vi "DependencyViewer_Configuration.vi"(8 "error in":errorcluster, 11 "ProjectPath":path) -> (0 "error out":errorcluster)   [LabVIEW 2020]
uses:
  <resource>/Framework/Providers/Open_GDS/DependencyViewer/DependencyChecker/FilterOptions.ctl
  <resource>/Framework/Providers/Open_GDS/SubVIs/GOOP_DependencySettings.ctl
  <resource>/Framework/Providers/Open_GDS/DependencyViewer/DependencyChecker/DependencyConfiguration.ctl
  <vilib>/Utility/sysdir.llb/System Directory Type.ctl
  <resource>/Framework/Providers/Open_GDS/DependencyViewer/DependencyChecker/DependencyChecker.lvlib
panel:
  in  "Max reports to save":u8 min=1
  in  "Close":bool
  in  "SaveChanges":bool
  in  "IgnoreLibrariesInCircularDependencies":bool
  in  "OnlyKeepCircularDepedencies":bool
  in  "Filter Options":T1={"Ignore user.lib"=FALSE, "Ignore vi.lib"=FALSE, "Ignore instr.lib"=FALSE, "FolderToIgnore"=[], "Ignore libraries"=FALSE, "Ignore lvcasses"=FALSE, "Ignore xnodes"=TRUE, "Ignore xcontrols"=TRUE, "Ignore Channel Classes"=TRUE}
  in  "RemoveEvenSubLibraries":bool
  in  "RemoveItemsBelongingToLibraries":bool
  in  "OpenFolder":bool
  in  "EmbedChartScript":bool
  in  "Remove Configuration":bool
  in  "Dependency configuration name":string
  in  "Add Configuration":bool
  in  "_ShowContextHelp":bool
  in  "Help":bool
  in  "Revert":bool
  in  "Update":bool
  out "ProductPicture":picture
  in  "Dependency configurations":i32(listbox) caption="Will show up in the right click menu"
  in  "UseProjectFolder":bool
  in  "Folder to save reports to":path
  # "Dependency Viewer Configuration"
  # "Filter option for configuration"
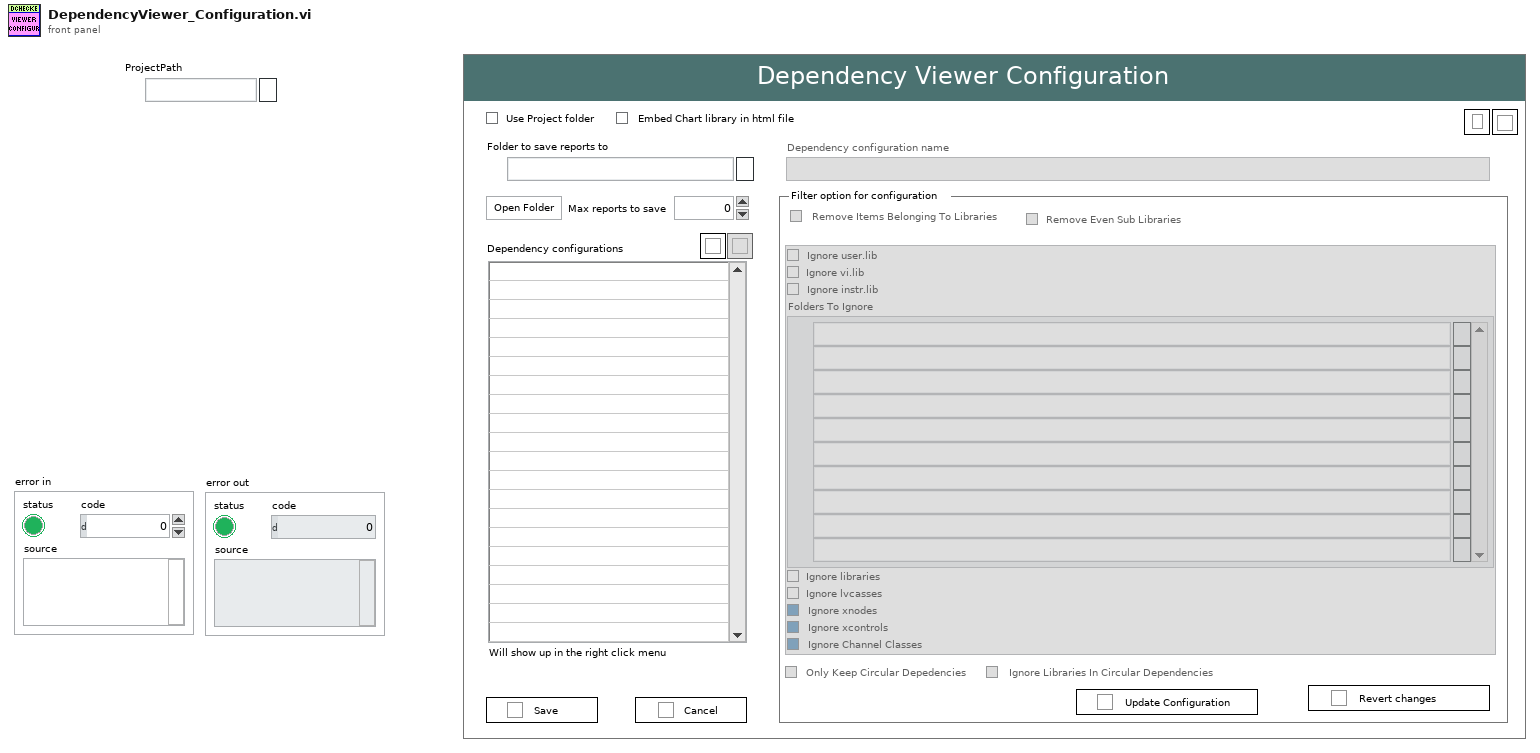
[diagram p1: front panel]
types:
  T1 = typedef "DependencyChecker.lvlib/FilterOptions.ctl" = cluster{"Ignore user.lib":bool, "Ignore vi.lib":bool, "Ignore instr.lib":bool, "FolderToIgnore":path[], "Ignore libraries":bool, "Ignore lvcasses":bool, "Ignore xnodes":bool, "Ignore xcontrols":bool, "Ignore Channel Classes":bool}
  T2 = typedef "System Directory Type.ctl" = i32
  T3 = typedef "GOOP_DependencySettings.ctl" = cluster{"EmbedChartLibraryScript":bool, "Configurations":T4[], "UseProjectFolder":bool, "Folder to save reports to":path, "Max reports to save":u8}
  T4 = typedef "DependencyChecker.lvlib/DependencyConfiguration.ctl" = cluster{"Name":string, "RemoveItemsBelongingToLibraries":bool, "RemoveEvenSubLibraries":bool, "FilterOptions":T1, "OnlyKeepCircularDepedencies":bool, "IgnoreLibrariesInCircularDependencies":bool}
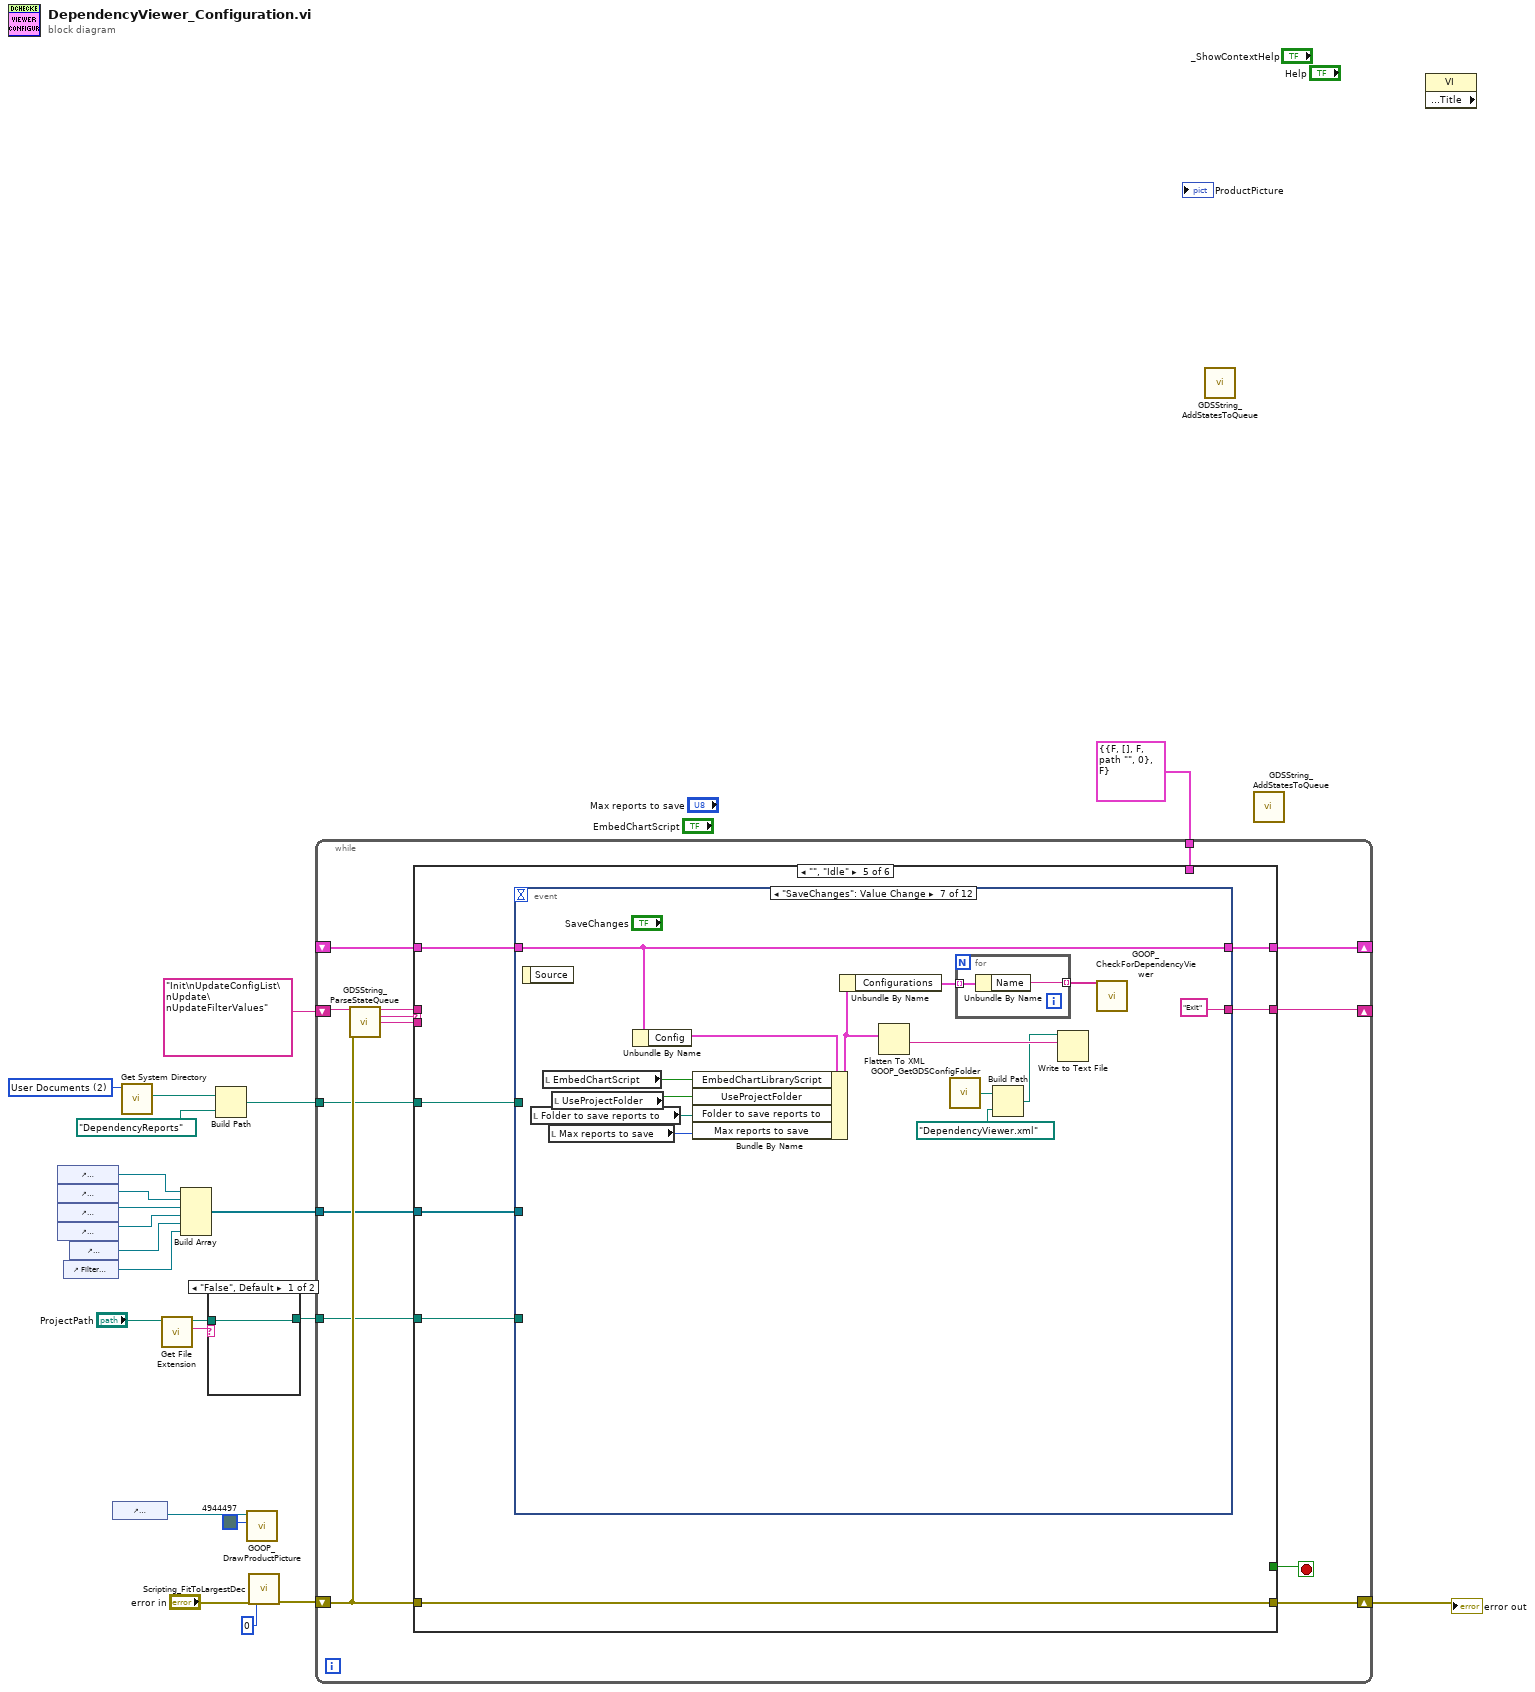
[diagram p0: block diagram]
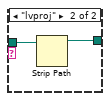
[diagram p2: hidden frame]
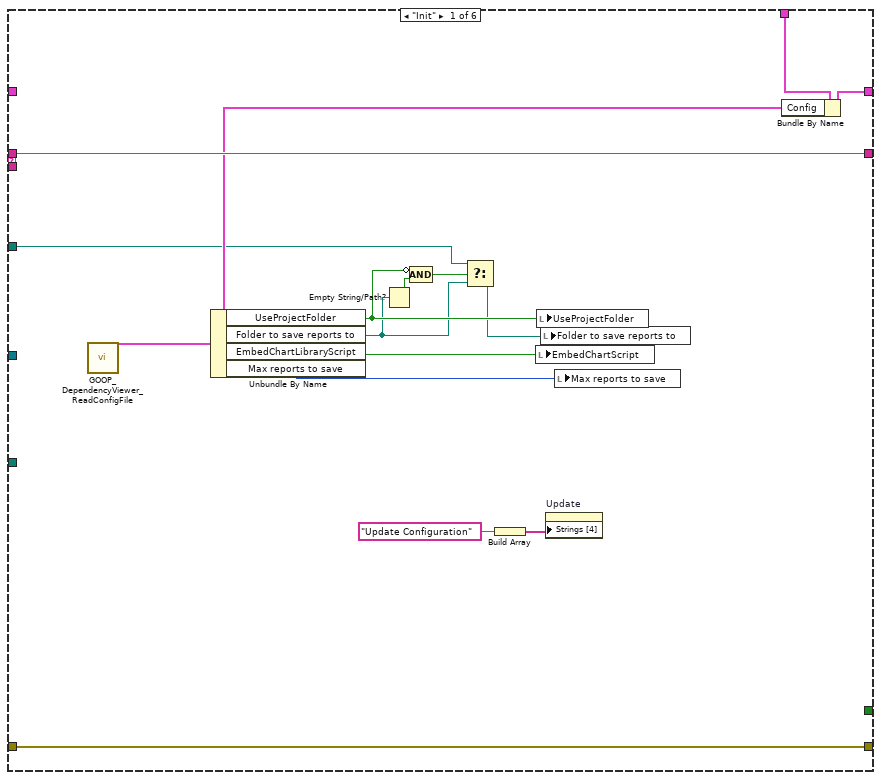
[diagram p3: hidden frame]
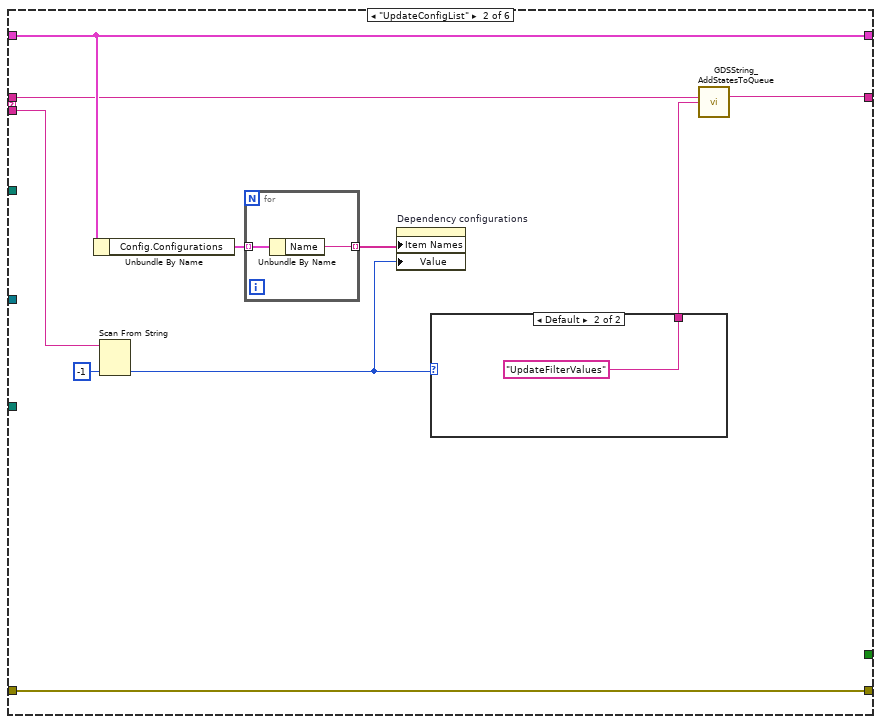
[diagram p4: hidden frame]
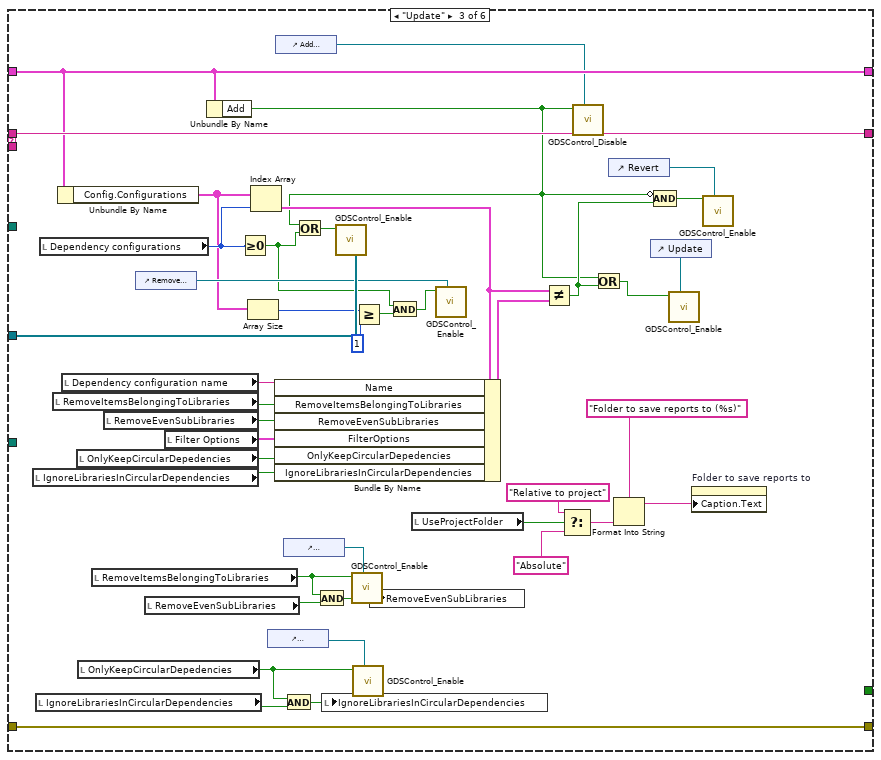
[diagram p6: hidden frame]
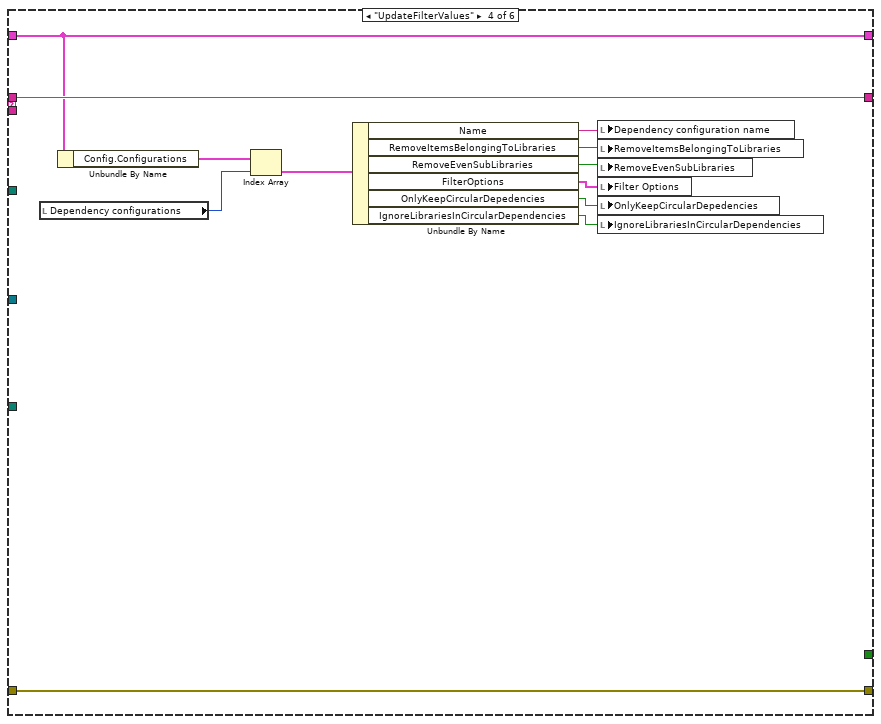
[diagram p7: hidden frame]
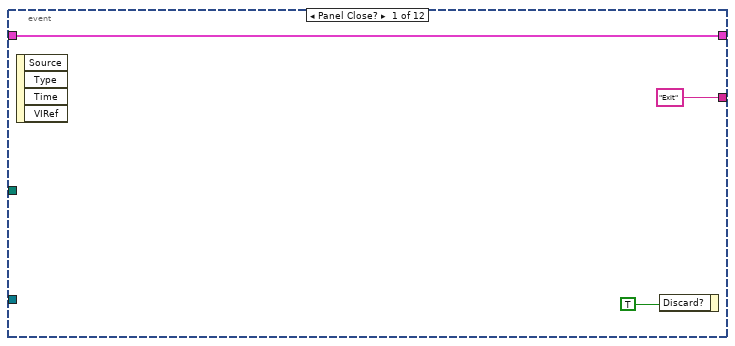
[diagram p8: hidden frame]
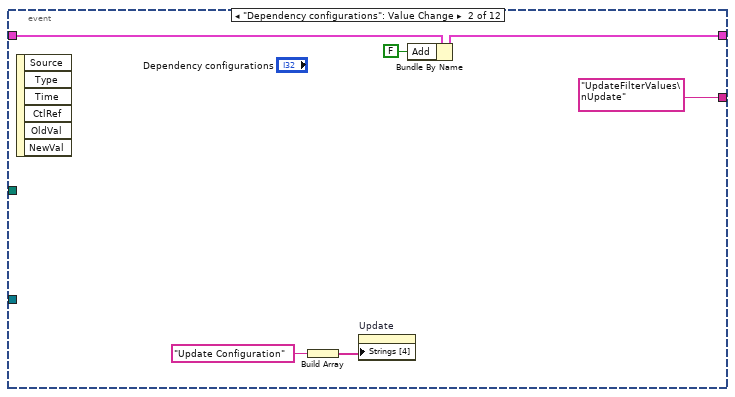
[diagram p9: hidden frame]
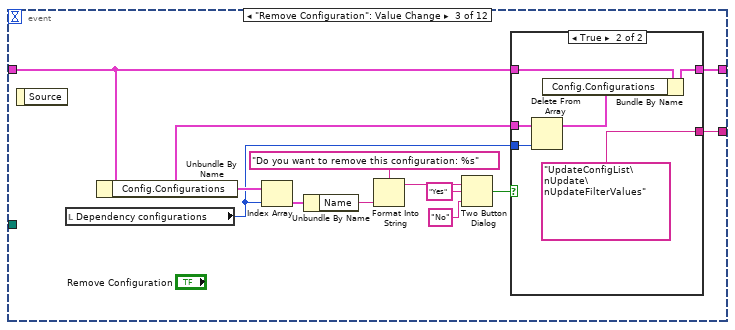
[diagram p10: hidden frame]
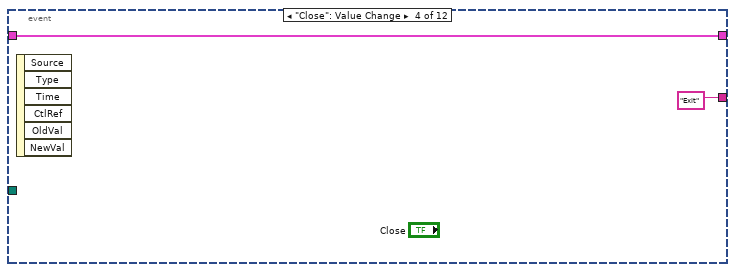
[diagram p12: hidden frame]
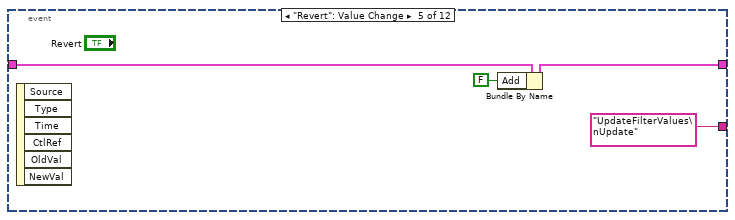
[diagram p13: hidden frame]
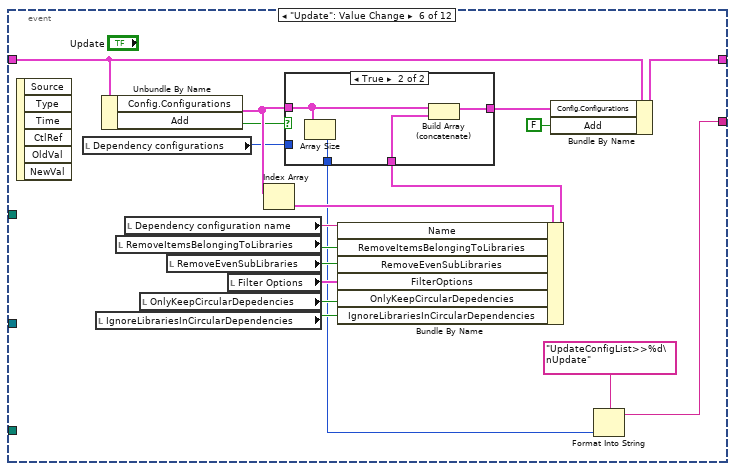
[diagram p14: hidden frame]
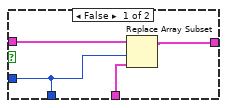
[diagram p15: hidden frame]
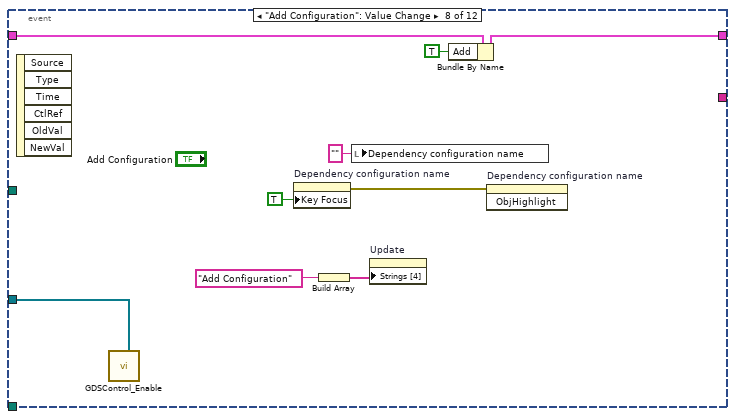
[diagram p16: hidden frame]
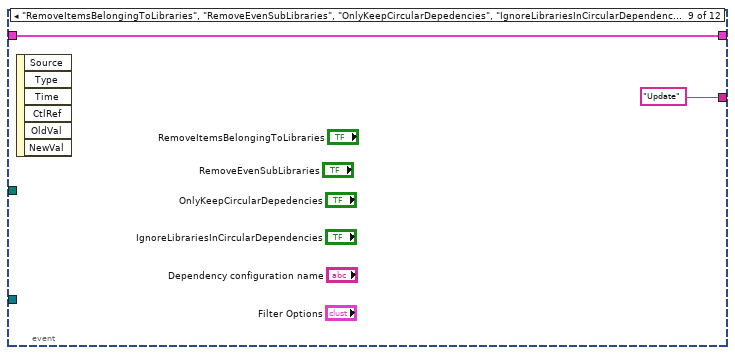
[diagram p17: hidden frame]
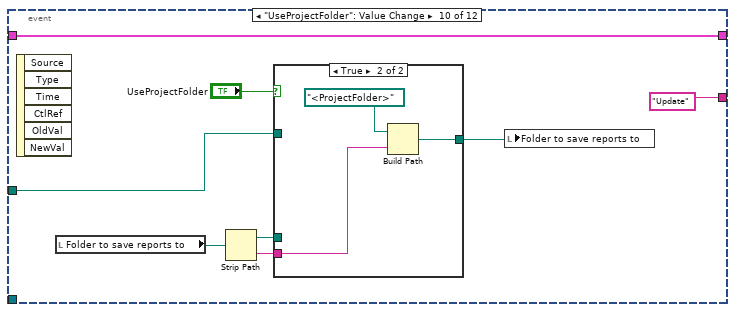
[diagram p18: hidden frame]
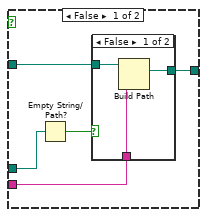
[diagram p19: hidden frame]
diagram:
  w8 = T2 2 items=["User Home"=0, "User Desktop"=1, "User Documents"=2, "User Application Data"=3, "User Preferences"=4, "User Temporary"=5, "Public Documents"=6, "Public Application Data"=7, "Public Preferences"=8, "Public Cache"=13, "System Core Libraries"=9, "System Installed Libraries"=10, "Application Files"=11, "Boot Volume Root"=12] ("system directory type")
  n1 = control-ref of="IgnoreLibrariesInCircularDependencies"() -> (w17:refnum<vi>)
  n2 = control-ref of="OnlyKeepCircularDepedencies"() -> (w16:refnum<vi>)
  n3 = control-ref of="RemoveEvenSubLibraries"() -> (w15:refnum<vi>)
  n4 = control-ref of="RemoveItemsBelongingToLibraries"() -> (w14:refnum<vi>)
  n5 = control-ref of="Filter Options"() -> (w12:refnum<vi>)
  n6 = control-ref of="Dependency configuration name"() -> (w13:refnum<vi>)
  n7 = control-ref of="ProductPicture"() -> (w22:refnum<vi>)
  n8 = call <vilib>:"Get System Directory.vi"("system directory type"=w8) -> ("system directory"=w7:path)  [unwired: 10 in]
  n9 = call <vilib>:"Get File Extension.vi"("file"="ProjectPath") -> ("lowercase file extension"=w3:string, "dup file"=w2:path)  [unwired: 6 in, 3 out]
  n10 = Build Array(w17, w16, w15, w14, w13, w12) -> (w11:refnum<vi>[])
  n11 = case shown="\"False\", Default" w3 {
    tunnel: w2 -> [w24 w26]
    tunnel: [w24 w25] -> w1
    frame "False", Default {
    }
    frame "lvproj" {
      n12 = Strip Path(path=w26) -> (stripped path=w25:path)  [unwired: 1 out]
    }
  }
  n13 = Build Path(base path=w7, name or relative path=path "DependencyReports") -> (appended path=w5:path)
  n14 = call <resource>:"GOOP_DrawProductPicture.vi"("BAckground ColorPane Color"=u32 4944497, "ProductPictureControl"=w22) -> ()  [unwired: 9 in, 1 out]
  n15 = call <resource>:"Scripting_FitToLargestDec.vi"("error in (no error)"="error in", "border spacing (2 px)"=0) -> ("error out"=w18:errorcluster)  [unwired: 4 in, 1 out]
  n16 = while {
    shift-right: [w35] -> _
    shift-left: "Init\nUpdateConfigList\nUpdate\nUpdateFilterValues" -> [w40]
    shift-right: [w37] -> w20
    shift-left: w18 -> [w38]
    tunnel: cluster{"Config":T3, "Add":bool} {"Config"={"EmbedChartLibraryScript"=FALSE, "Configurations"=[], "UseProjectFolder"=FALSE, "Folder to save reports to"=path "", "Max reports to save"=0}, "Add"=FALSE} -> [w33]
    shift-right: [w32] -> _
    shift-left: _ -> [w31]
    tunnel: w11 -> [w29]
    tunnel: w5 -> [w28]
    tunnel: w1 -> [w27]
    stop <- w34 stop-if-true
    n17 = call <resource>:"GDSString_ParseStateQueue.vi"("State Queue"=w40, "Error In (no error)"=w38) -> ("Remaining States"=w36:string, "Current State"=w39:string, "Arguments"=w30:string)  [unwired: 9 in, 2 out]
    n18 = case shown="\"\", \"Idle\"" w39 {
      tunnel: w38 -> [w55 w65 w101 w121 w129 w265]
      tunnel: [w55 w65 w101 w121 w129 w265] -> w37
      tunnel: [w54 w58 w102 w122 w126 w267] -> w35
      tunnel: w36 -> [w54 w59 w102 w122 _ w267]
      tunnel: [_ _ _ _ _ TRUE] -> w34
      tunnel: w33 -> [w53 _ _ _ _ _]
      tunnel: [w52 w63 w83 w120 w127 w264] -> w32
      tunnel: w31 -> [_ w63 w83 w120 w128 w264]
      tunnel: w30 -> [_ w61 _ _ _ _]
      tunnel: w29 -> [_ _ w99 _ w123 _]
      tunnel: w28 -> [w41 _ _ _ w125 _]
      tunnel: w27 -> [_ _ _ _ w124 _]
      frame "Init" {
        n19 = call <resource>:"GOOP_DependencyViewer_ReadConfigFile.vi"() -> ("Config"=w51:T3)  [unwired: 11 in]
        n20 = Unbundle By Name(w51) -> ("UseProjectFolder"=w46:bool, "Folder to save reports to"=w43:path, "EmbedChartLibraryScript"=w50:bool, "Max reports to save"=w47:u8)
        n21 = Empty String/Path?(string/path=w43) -> (empty?=w45:bool)
        n22 = Compound Arithmetic op=AND(invert w46, w45) -> (w44:bool)
        n23 = Select(t=w41, s=w44, f=w43) -> (s? t:f=w42:path)
        n24 = Build Array("Update Configuration") -> (w49:string[])
        n25 = local write "EmbedChartScript"(w50) -> ()
        n26 = local write "UseProjectFolder"(w46) -> ()
        n27 = local write "Folder to save reports to"(w42) -> ()
        n28 = property on="Update" class="Bool"("Strings [4]"=w49) -> ()  [unwired: 2 in, 2 out]
        n29 = local write "Max reports to save"(w47) -> ()
        n30 = Bundle By Name(cluster=w53, "Config"=w51) -> (w52:cluster{"Config":T3, "Add":bool})
      }
      frame "UpdateConfigList" {
        n31 = Unbundle By Name(w63) -> ("Config.Configurations"=w64:T4[])
        n32 = Scan From String(input string=w61, default 1=-1 ("default value 1")) -> (output 1=w57:i32)  [unwired: 3 in, 3 out]
        n33 = for {
          tunnel: w64 -> [w68] mode=indexing
          tunnel: [w67] -> w62 mode=indexing
          n34 = Unbundle By Name(w68) -> ("Name"=w67:string)
        }
        n35 = property on="Dependency configurations" class="LstBox (strict)"("Item Names"=w62, "Value"=w57) -> ()  [unwired: 2 in, 2 out]
        n36 = case shown="Default" w57 {
          tunnel: [_ "UpdateFilterValues"] -> w56
          frame -1 {
          }
          frame Default {
          }
        }
        n37 = call <resource>:"GDSString_AddStatesToQueue.vi"("State(s) in (\"\")"=w59, "State(s) at Back (\"\")"=w56) -> ("States Out"=w58:string)  [unwired: 13 in]
      }
      frame "Update" {
        n38 = local read "IgnoreLibrariesInCircularDependencies"() -> (w92:bool)
        n39 = local read "IgnoreLibrariesInCircularDependencies"() -> (w104:bool)
        n40 = local read "Dependency configurations"() -> (w100:i32)
        n41 = local read "RemoveItemsBelongingToLibraries"() -> (w96:bool)
        n42 = Unbundle By Name(w83) -> ("Config.Configurations"=w89:T4[])
        n43 = local read "Dependency configuration name"() -> (w97:string)
        n44 = local read "OnlyKeepCircularDepedencies"() -> (w93:bool)
        n45 = local read "OnlyKeepCircularDepedencies"() -> (w105:bool)
        n46 = local read "RemoveItemsBelongingToLibraries"() -> (w108:bool)
        n47 = local read "RemoveEvenSubLibraries"() -> (w95:bool)
        n48 = control-ref of="Remove Configuration"() -> (w98:refnum<vi>)
        n49 = local read "RemoveEvenSubLibraries"() -> (w109:bool)
        n50 = local read "Filter Options"() -> (w94:T1)
        n51 = Unbundle By Name(w83) -> ("Add"=w70:bool)
        n52 = Greater Or Equal To 0?(x=w100) -> (x >= 0?=w74:bool)
        n53 = Array Size(array=w89) -> (size(s)=w88:i32)
        n54 = Index Array(array=w89, index=w100) -> (element=w90:T4)
        n55 = control-ref of="IgnoreLibrariesInCircularDependencies"() -> (w106:refnum<vi>)
        n56 = Bundle By Name(cluster=w90, "Name"=w97, "RemoveItemsBelongingToLibraries"=w96, "RemoveEvenSubLibraries"=w95, "FilterOptions"=w94, "OnlyKeepCircularDepedencies"=w93, "IgnoreLibrariesInCircularDependencies"=w92) -> (w91:T4)
        n57 = control-ref of="Add Configuration"() -> (w69:refnum<vi>)
        n58 = control-ref of="RemoveEvenSubLibraries"() -> (w110:refnum<vi>)
        n59 = And(x=w105, y=w104) -> (x .and. y?=w103:bool)
        n60 = Or(x=w70, y=w74) -> (x .or. y?=w73:bool)
        n61 = And(x=w108, y=w109) -> (x .and. y?=w107:bool)
        n62 = local write "IgnoreLibrariesInCircularDependencies"(w103) -> ()
        n63 = call <resource>:"GDSControl_Enable.vi"("ManyControls"=w99, "Enable(True)"=w73) -> ()  [unwired: 9 in, 1 out]
        n64 = call <resource>:"GDSControl_Enable.vi"("ControlRefnum(IgnoreIfNotWired)"=w110, "Enable(True)"=w108) -> ()  [unwired: 9 in, 1 out]
        n65 = call <resource>:"GDSControl_Enable.vi"("ControlRefnum(IgnoreIfNotWired)"=w106, "Enable(True)"=w105) -> ()  [unwired: 9 in, 1 out]
        n66 = Greater Or Equal?(x=w88, y=1) -> (x >= y?=w86:bool)
        n67 = local write "RemoveEvenSubLibraries"(w107) -> ()
        n68 = And(x=w74, y=w86) -> (x .and. y?=w85:bool)
        n69 = local read "UseProjectFolder"() -> (w79:bool)
        n70 = call <resource>:"GDSControl_Enable.vi"("ControlRefnum(IgnoreIfNotWired)"=w98, "Enable(True)"=w85) -> ()  [unwired: 9 in, 1 out]
        n71 = Not Equal?(x=w90, y=w91) -> (x != y?=w72:bool)
        n72 = Select(t="Relative to project", s=w79, f="Absolute") -> (s? t:f=w78:string)
        n73 = call <resource>:"GDSControl_Disable.vi"("ControlRefnum(IgnoreIfNotWired)"=w69, "Disasble(True)"=w70) -> ()  [unwired: 9 in, 1 out]
        n74 = Or(x=w70, y=w72) -> (x .or. y?=w71:bool)
        n75 = control-ref of="Revert"() -> (w81:refnum<vi>)
        n76 = Format Into String(format string="Folder to save reports to (%s)", w78) -> (resulting string=w77:string)  [unwired: 2 in, 1 out]
        n77 = control-ref of="Update"() -> (w84:refnum<vi>)
        n78 = Compound Arithmetic op=AND(invert w70, w72) -> (w82:bool)
        n79 = call <resource>:"GDSControl_Enable.vi"("ControlRefnum(IgnoreIfNotWired)"=w84, "Enable(True)"=w71) -> ()  [unwired: 9 in, 1 out]
        n80 = property on="Folder to save reports to" class="Path"("Caption.Text"=w77) -> ()  [unwired: 2 in, 2 out]
        n81 = call <resource>:"GDSControl_Enable.vi"("ControlRefnum(IgnoreIfNotWired)"=w81, "Enable(True)"=w82) -> ()  [unwired: 9 in, 1 out]
      }
      frame "UpdateFilterValues" {
        n82 = local read "Dependency configurations"() -> (w118:i32)
        n83 = Unbundle By Name(w120) -> ("Config.Configurations"=w119:T4[])
        n84 = Index Array(array=w119, index=w118) -> (element=w117:T4)
        n85 = Unbundle By Name(w117) -> ("Name"=w116:string, "RemoveItemsBelongingToLibraries"=w115:bool, "RemoveEvenSubLibraries"=w114:bool, "FilterOptions"=w113:T1, "OnlyKeepCircularDepedencies"=w112:bool, "IgnoreLibrariesInCircularDependencies"=w111:bool)
        n86 = local write "Dependency configuration name"(w116) -> ()
        n87 = local write "RemoveItemsBelongingToLibraries"(w115) -> ()
        n88 = local write "RemoveEvenSubLibraries"(w114) -> ()
        n89 = local write "Filter Options"(w113) -> ()
        n90 = local write "OnlyKeepCircularDepedencies"(w112) -> ()
        n91 = local write "IgnoreLibrariesInCircularDependencies"(w111) -> ()
      }
      frame "", "Idle" {
        n92 = event shown="[6] \"SaveChanges\": Value Change" {
          selector: _ -> [_ _ _ _ _ _ _ _ _ _ _ _]
          dyn-events: _ -> [_ _ _ _ _ _ _ _ _ _ _ _]
          timeout: _ -> [_ _ _ _ _ _ _ _ _ _ _ _]
          tunnel: w128 -> [w132 w137 w141 w159 w163 w175 w202 w214 w216 w224 w244 w260]
          tunnel: [w132 w134 w143 w159 w161 w174 w202 w210 w216 w224 w244 w260] -> w127
          tunnel: ["Exit" "UpdateFilterValues\nUpdate" w139 "Exit" "UpdateFilterValues\nUpdate" w165 "Exit" _ "Update" "Update" _ _] -> w126
          tunnel: w125 -> [_ _ _ _ _ _ _ _ _ w218 _ _]
          tunnel: w124 -> [_ _ _ _ _ _ _ _ _ _ w239 _]
          tunnel: w123 -> [_ _ _ _ _ _ _ w211 _ _ _ _]
          event Panel Close? {
            n93 = event-data() -> ()  [unwired: 1 in, 4 out]
            n94 = event-data("Discard?"=TRUE) -> ()  [unwired: 1 in, 1 out]
          }
          event "Dependency configurations": Value Change {
            n95 = event-data() -> ()  [unwired: 1 in, 6 out]
            n96 = Build Array("Update Configuration") -> (w136:string[])
            n97 = property on="Update" class="Bool"("Strings [4]"=w136) -> ()  [unwired: 2 in, 2 out]
            n98 = Bundle By Name(cluster=w137, "Add"=FALSE) -> (w134:cluster{"Config":T3, "Add":bool})
          }
          event "Remove Configuration": Value Change {
            n99 = event-data() -> ()  [unwired: 1 in, 1 out]
            n100 = local read "Dependency configurations"() -> (w140:i32)
            n101 = Unbundle By Name(w141) -> ("Config.Configurations"=w142:T4[])
            n102 = Index Array(array=w142, index=w140) -> (element=w150:T4)
            n103 = Unbundle By Name(w150) -> ("Name"=w148:string)
            n104 = Format Into String(format string="Do you want to remove this configuration: %s", w148) -> (resulting string=w147:string)  [unwired: 2 in, 1 out]
            n105 = Two Button Dialog(message=w147, 1:"No" ("T button name (\"OK\")"), 2:"Yes" ("T button name (\"OK\")")) -> (T button?=w144:bool)
            n106 = case shown="True" w144 {
              tunnel: [w151 w154] -> w143
              tunnel: w142 -> [_ w157]
              tunnel: w141 -> [w151 w156]
              tunnel: w140 -> [_ w153]
              tunnel: [_ "UpdateConfigList\nUpdate\nUpdateFilterValues"] -> w139
              frame False {
              }
              frame True {
                n107 = Delete From Array(array=w157, index=w153) -> (array with subset deleted=w155:T4[])  [unwired: 1 in, 1 out]
                n108 = Bundle By Name(cluster=w156, "Config.Configurations"=w155) -> (w154:cluster{"Config":T3, "Add":bool})
              }
            }
          }
          event "Close": Value Change {
            n109 = event-data() -> ()  [unwired: 1 in, 6 out]
          }
          event "Revert": Value Change {
            n110 = event-data() -> ()  [unwired: 1 in, 6 out]
            n111 = Bundle By Name(cluster=w163, "Add"=FALSE) -> (w161:cluster{"Config":T3, "Add":bool})
          }
          event "Update": Value Change {
            n112 = event-data() -> ()  [unwired: 1 in, 6 out]
            n113 = local read "Dependency configurations"() -> (w168:i32)
            n114 = local read "IgnoreLibrariesInCircularDependencies"() -> (w176:bool)
            n115 = Unbundle By Name(w175) -> ("Config.Configurations"=w171:T4[], "Add"=w169:bool)
            n116 = local read "RemoveItemsBelongingToLibraries"() -> (w180:bool)
            n117 = local read "Dependency configuration name"() -> (w181:string)
            n118 = local read "OnlyKeepCircularDepedencies"() -> (w177:bool)
            n119 = local read "RemoveEvenSubLibraries"() -> (w179:bool)
            n120 = local read "Filter Options"() -> (w178:T1)
            n121 = Index Array(array=w171) -> (element=w170:T4)  [unwired: 1 in]
            n122 = Bundle By Name(cluster=w170, "Name"=w181, "RemoveItemsBelongingToLibraries"=w180, "RemoveEvenSubLibraries"=w179, "FilterOptions"=w178, "OnlyKeepCircularDepedencies"=w177, "IgnoreLibrariesInCircularDependencies"=w176) -> (w173:T4)
            n123 = case shown="True" w169 {
              tunnel: w173 -> [w183 w189]
              tunnel: [w184 w188] -> w172
              tunnel: w171 -> [w185 w187]
              tunnel: w168 -> [w182 _]
              tunnel: [w182 w186] -> w164
              frame False {
                n124 = Replace Array Subset(array=w185, new element=w183, index=w182) -> (w184:T4[])
              }
              frame True {
                n125 = Array Size(array=w187) -> (size(s)=w186:i32)
                n126 = Build Array (concatenate)(w187, w189) -> (w188:T4[])
              }
            }
            n127 = Bundle By Name(cluster=w175, "Config.Configurations"=w172, "Add"=FALSE) -> (w174:cluster{"Config":T3, "Add":bool})
            n128 = Format Into String(format string="UpdateConfigList>>%d\nUpdate", w164) -> (resulting string=w165:string)  [unwired: 2 in, 1 out]
          }
          event "SaveChanges": Value Change {
            n129 = event-data() -> ()  [unwired: 1 in, 1 out]
            n130 = local read "Folder to save reports to"() -> (w191:path)
            n131 = local read "EmbedChartScript"() -> (w193:bool)
            n132 = local read "Max reports to save"() -> (w190:u8)
            n133 = local read "UseProjectFolder"() -> (w192:bool)
            n134 = Unbundle By Name(w202) -> ("Config"=w197:T3)
            n135 = Bundle By Name(cluster=w197, "EmbedChartLibraryScript"=w193, "UseProjectFolder"=w192, "Folder to save reports to"=w191, "Max reports to save"=w190) -> (w196:T3)
            n136 = Unbundle By Name(w196) -> ("Configurations"=w195:T4[])
            n137 = Flatten To XML(6:w196) -> (2:w199:string)
            n138 = call <resource>:"GOOP_GetGDSConfigFolder.vi"() -> ("GDSFolderPath"=w201:path)
            n139 = for {
              tunnel: [w205] -> w194 mode=indexing
              tunnel: w195 -> [w204] mode=indexing
              n140 = Unbundle By Name(w204) -> ("Name"=w205:string)
            }
            n141 = Build Path(base path=w201, name or relative path=path "DependencyViewer.xml") -> (appended path=w198:path)
            n142 = Write to Text File(file (use dialog)=w198, text=w199) -> ()  [unwired: 2 in, 3 out]
            n143 = call <resource>:"GOOP_CheckForDependencyViewer.vi"("Configurations"=w194) -> ()  [unwired: 8 in, 3 out]
          }
          event "Add Configuration": Value Change {
            n144 = event-data() -> ()  [unwired: 1 in, 6 out]
            n145 = call <resource>:"GDSControl_Enable.vi"("ManyControls"=w211) -> ()  [unwired: 10 in, 1 out]
            n146 = property on="Dependency configuration name" class="Str"("Key Focus"=TRUE ("Add")) -> (error out=w206:errorcluster)  [unwired: 2 in, 1 out]
            n147 = Build Array("Add Configuration") -> (w213:string[])
            n148 = local write "Dependency configuration name"("" ("Dependency configuration name")) -> ()
            n149 = property on="Update" class="Bool"("Strings [4]"=w213) -> ()  [unwired: 2 in, 2 out]
            n150 = Bundle By Name(cluster=w214, "Add"=TRUE) -> (w210:cluster{"Config":T3, "Add":bool})
            n151 = invoke on="Dependency configuration name" class="Str" method="ObjHighlight"(error in=w206) -> ()  [unwired: 2 in, 3 out]
          }
          event "RemoveItemsBelongingToLibraries", "RemoveEvenSubLibraries", "OnlyKeepCircularDepedencies", "IgnoreLibrariesInCircularDependencies", "Dependency configuration name": Value Change {
            n152 = event-data() -> ()  [unwired: 1 in, 6 out]
          }
          event "UseProjectFolder": Value Change {
            n153 = event-data() -> ()  [unwired: 1 in, 6 out]
            n154 = local read "Folder to save reports to"() -> (w221:path)
            n155 = Strip Path(path=w221) -> (stripped path=w217:path, name=w220:string)
            n156 = case shown="True" "UseProjectFolder" {
              tunnel: w220 -> [w225 w235]
              tunnel: [w226 w234] -> w219
              tunnel: w218 -> [w229 _]
              tunnel: w217 -> [w228 _]
              frame False {
                n157 = Empty String/Path?(string/path=w228) -> (empty?=w227:bool)
                n158 = case shown="False" w227 {
                  tunnel: w229 -> [w232 w233]
                  tunnel: [w230 w233] -> w226
                  tunnel: w225 -> [w231 _]
                  frame False {
                    n159 = Build Path(base path=w232, name or relative path=w231) -> (appended path=w230:path)
                  }
                  frame True {
                  }
                }
              }
              frame True {
                n160 = Build Path(base path=path "<ProjectFolder>", name or relative path=w235) -> (appended path=w234:path)
              }
            }
            n161 = local write "Folder to save reports to"(w219) -> ()
          }
          event "OpenFolder": Value Change {
            n162 = event-data() -> ()  [unwired: 1 in, 6 out]
            n163 = local read "Folder to save reports to"() -> (w241:path)
            n164 = local read "UseProjectFolder"() -> (w242:bool)
            n165 = case shown="True" w242 {
              tunnel: w241 -> [w245 w249]
              tunnel: [w245 w246] -> w238
              tunnel: w239 -> [_ w248]
              frame False {
              }
              frame True {
                n166 = Strip Path(path=w249) -> (name=w247:string)  [unwired: 1 out]
                n167 = Build Path(base path=w248, name or relative path=w247) -> (appended path=w246:path)
              }
            }
            n168 = call <vilib>:"Create Directory Recursive.vi"("directory"=w238) -> ("directory copy"=w237:path)  [unwired: 4 in, 2 out]
            n169 = Format Into String(format string="explorer \"%s\"", w237) -> (resulting string=w240:string)  [unwired: 2 in, 1 out]
            n170 = call <vilib>:"System Exec.vi"("command line"=w240) -> ()  [unwired: 7 in, 4 out]
          }
          event "Folder to save reports to": Value Change {
            n171 = event-data() -> ()  [unwired: 1 in, 6 out]
            n172 = Path Type(1:"Folder to save reports to") -> (0:w257:i16)
            n173 = Strip Path(path="Folder to save reports to") -> (name=w259:string)  [unwired: 1 out]
            n174 = Equal?(x=w257, y=i16 1) -> (x = y?=w253:bool)
            n175 = Match Pattern(string=w259, regular expression="<") -> (offset past match=w255:i32)  [unwired: 1 in, 3 out]
            n176 = Greater Or Equal To 0?(x=w255) -> (x >= 0?=w252:bool)
            n177 = Compound Arithmetic op=AND(w253, invert w252) -> (w251:bool)
            n178 = Or(x=w253, y=w252) -> (x .or. y?=w254:bool)
            n179 = case shown="True" w251 {
              tunnel: "Folder to save reports to" -> [_ w262]
              frame False {
              }
              frame True {
                n180 = Build Path(base path=path "<ProjectFolder>", name or relative path=w262) -> (appended path=w261:path)
                n181 = local write "Folder to save reports to"(w261) -> ()
              }
            }
            n182 = local write "UseProjectFolder"(w254) -> ()
          }
        }
      }
      frame "Error", "Exit", Default {
      }
    }
  }
  "error out" <- w20
  n183 = call <resource>:"GDSString_AddStatesToQueue.vi"() -> ()  [unwired: 15 in, 1 out]
  n184 = call <resource>:"GDSString_AddStatesToQueue.vi"() -> ()  [unwired: 15 in, 1 out]
  n185 = property class="VI" props=["Front Panel.Title"]() -> ()  [unwired: 2 in, 3 out]
